vi "logsSD.vi"(2 "error in (no error)":errorcluster, 3 "Real delay time, ps":dbl, 4 "Log":bool, 5 "Experiment in":refnum<class "Experiment.lvclass">) -> (0 "error out":errorcluster, 1 "Path":path)   [LabVIEW 2015]
uses:
  Classes/Experiment.lvclass
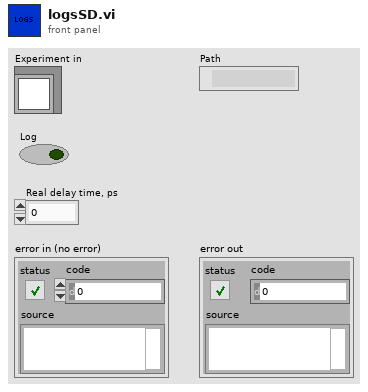
[diagram p1: front panel]
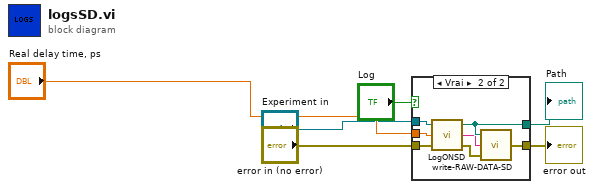
[diagram p0: block diagram]
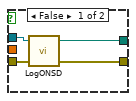
[diagram p2: hidden frame]
diagram:
  n1 = case shown="Vrai" "Log" {
    tunnel: "error in (no error)" -> [w8 w17]
    tunnel: [w9 w16] -> w4
    tunnel: "Experiment in" -> [w10 w15]
    tunnel: [w7 w11] -> w2
    tunnel: "Real delay time, ps" -> [_ w14]
    frame False {
      n2 = call "LogONSD.vi"("error in (no error)"=w8, "Experiment in"=w10) -> ("error out"=w7:errorcluster, "Path"=w9:path)  [unwired: 1 in, 1 out]
    }
    frame True {
      n3 = call "LogONSD.vi"("error in (no error)"=w17, "Real delay time, ps"=w14, "Experiment in"=w15) -> ("error out"=w12:errorcluster, "String"=w13:string, "Path"=w16:path)
      n4 = call "write-RAW-DATA-SD.vi"("error in (no error)"=w12, "Text"=w13, "File"=w16) -> ("error out"=w11:errorcluster)
    }
  }
  "Path" <- w4
  "error out" <- w2
